vi "GetSystemDefinitionPropertyValue_I16.vi"(8 "error in (no error)":errorcluster, 10 "property name":string, 11 "BaseNodeType in":refnum<k39>) -> (0 "error out":errorcluster, 2 "value":i16, 3 "BaseNodeType out":refnum<k39>)   [LabVIEW 2027, in "VeriStandTestUtilities.lvlib"]
uses:
  VeriStandTestUtilities.lvlib
  C:/NetCoreDLL/NationalInstruments.VeriStand.SystemStorage.dll
  NetCoreDLL/NationalInstruments.VeriStand.SystemStorage.dll
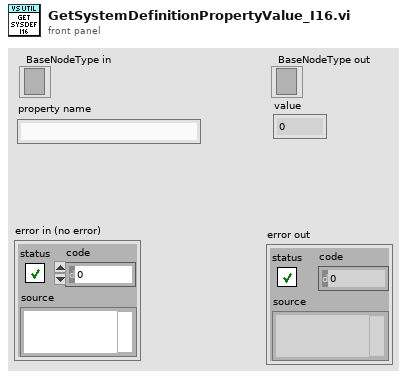
[diagram p1: front panel]
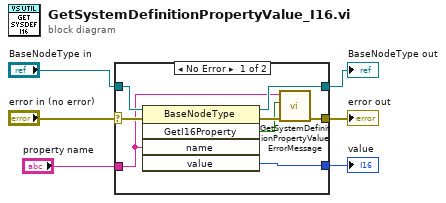
[diagram p0: block diagram]
diagram:
  n1 = case shown="No Error" "error in (no error)" {
    selector: "error in (no error)" -> [w13 w16]
    tunnel: "BaseNodeType in" -> [w14 w15]
    tunnel: "property name" -> [w8 _]
    tunnel: [w12 w15] -> w3
    tunnel: [w9 w16] -> w2
    tunnel: [w11 _] -> w1
    frame No Error {
      n2 = invoke class="BaseNodeType" method="GetI16Property"(reference=w14, error in=w13, "name"=w8) -> (reference out=w12:refnum<k39>, error out=w10:errorcluster, "GetI16Property"=w7:bool, "value"=w11:i16)  [unwired: 2 in, 1 out]
      n3 = call "GetSystemDefinitionPropertyValueErrorMessage.vi"("error in (no error)"=w10, "successful?"=w7, "property name"=w8) -> ("error out"=w9:errorcluster)  [unwired: 8 in]
    }
    frame Error {
    }
  }
  "error out" <- w2
  "BaseNodeType out" <- w3
  "value" <- w1
